vi "Read byte.vi"(8 "error in":errorcluster, 11 "Profibus channel in":refnum<class "Profibus channel.lvclass">) -> (0 "error out":errorcluster, 2 "byte":i32, 3 "Profibus channel out":refnum<class "Profibus channel.lvclass">)   [LabVIEW 2013, in "Profibus channel.lvclass"]
uses:
  Profibus channel.lvclass
  Profibus channel.lvclass/Profibus channel.ctl
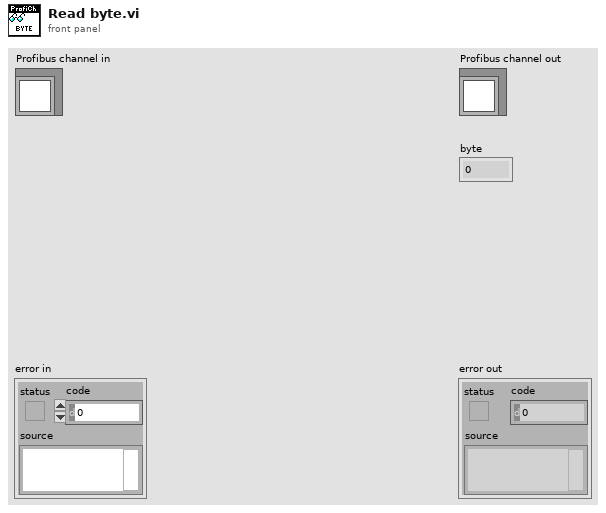
[diagram p1: front panel]
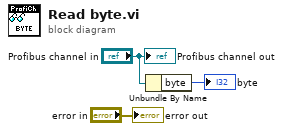
[diagram p0: block diagram]
diagram:
  n1 = Unbundle By Name("Profibus channel in") -> ("byte"=→"byte":i32)
  "error out" <- "error in"
  "Profibus channel out" <- "Profibus channel in"
